vi "LoopThroughTab.vi"() -> ()   [LabVIEW 2019]
uses:
  <vilib>/Utility/file.llb/Write Delimited Spreadsheet (string).vi
panel:
  out "Value Array":dbl[](array[numeric])
  in  "Numeric 9":dbl
  in  "Numeric 8":dbl
  in  "Numeric 7":dbl
  in  "Numeric 6":dbl
  in  "Numeric 5":dbl
  out "Label Array":string[](array[string])
  in  "Tab Control":enum32{"Page 1", "Page 2"}(tab)
  in  "Numeric 10":dbl
  in  "Numeric 4":dbl
  in  "Numeric 3":dbl
  in  "Numeric 2":dbl
  in  "Numeric":dbl
  in  "String":string
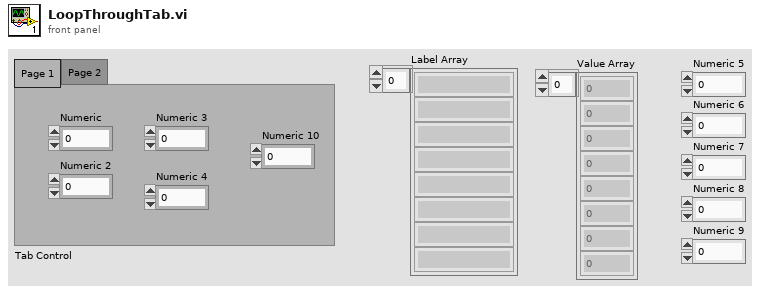
[diagram p1: front panel]
types:
  T1 = enum16{"open", "replace", "create", "open or create", "replace or create", "replace or create with confirmation"}
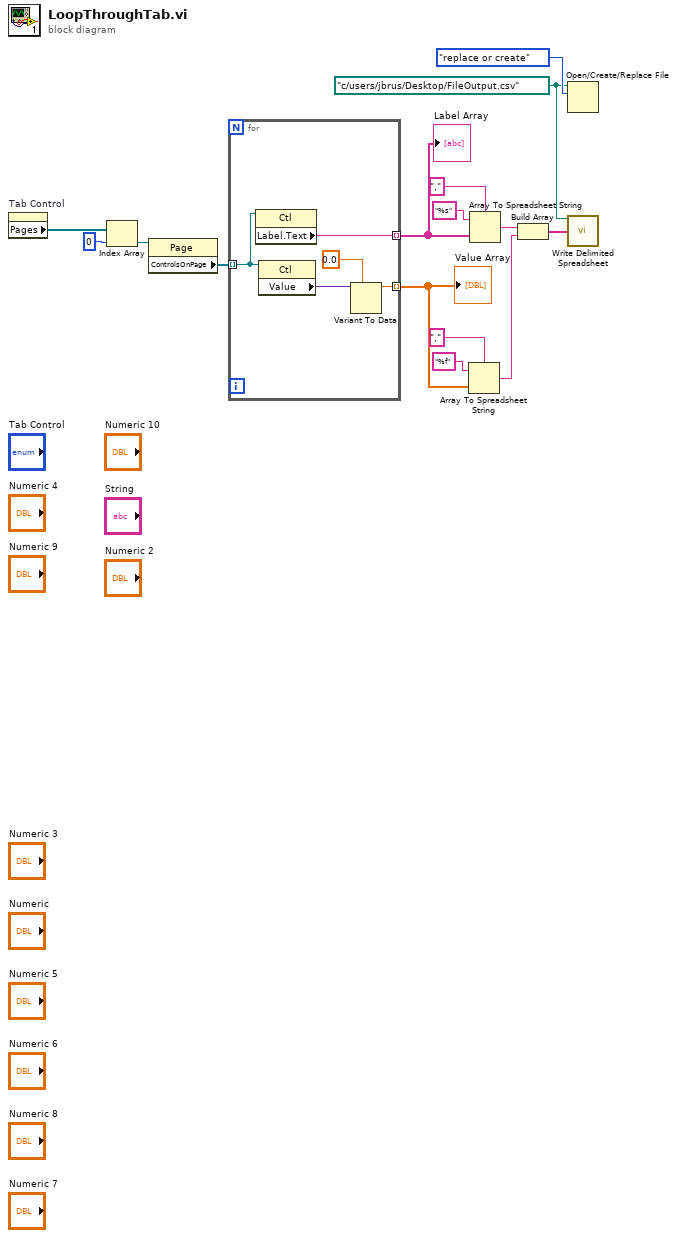
[diagram p0: block diagram]
diagram:
  w5 = path "c:/users/jbrus/Desktop/FileOutput.csv" ("file path (dialog if empty)")
  n1 = property on="Tab Control" class="TabCtl (strict)"() -> ("Pages"=w15:refnum<vi>[])  [unwired: 2 in, 2 out]
  n2 = Index Array(array=w15, index=0) -> (element=w13:refnum<vi>)
  n3 = property class="Page"(reference=w13) -> ("ControlsOnPage"=w12:refnum<vi>[])  [unwired: 1 in, 2 out]
  n4 = for {
    tunnel: w12 -> [w19] mode=indexing
    tunnel: [w20] -> w6 mode=indexing
    tunnel: [w16] -> w4 mode=indexing
    n5 = property class="Ctl"(reference=w19) -> ("Label.Text"=w20:string)  [unwired: 1 in, 2 out]
    n6 = property class="Ctl"(reference=w19) -> ("Value"=w18:variant)  [unwired: 1 in, 2 out]
    n7 = Variant To Data(type=0.0, Variant=w18) -> (data=w16:dbl)  [unwired: 1 in, 1 out]
  }
  "Label Array" <- w6
  "Value Array" <- w4
  n8 = Array To Spreadsheet String(delimiter (Tab)=",", array=w4, 3:"%f" ("format string")) -> (spreadsheet string=w3:string)
  n9 = Array To Spreadsheet String(delimiter (Tab)=",", array=w6, 3:"%s" ("format string")) -> (spreadsheet string=w1:string)
  n10 = Build Array(w1, w3) -> (w2:string[])
  n11 = Open/Create/Replace File(file path (use dialog)=w5, operation (0:open)=T1."replace or create") -> ()  [unwired: 4 in, 3 out]
  n12 = call-poly <vilib>:"Write Delimited Spreadsheet.vi"("file path (dialog if empty)"=w5, "1D data"=w2) -> ()  [unwired: 12 in, 2 out]
